vi "abort_delta.vi"() -> ()   [LabVIEW 2019]
panel:
  in  "Abort Conductance":bool
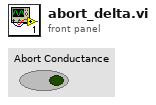
[diagram p1: front panel]
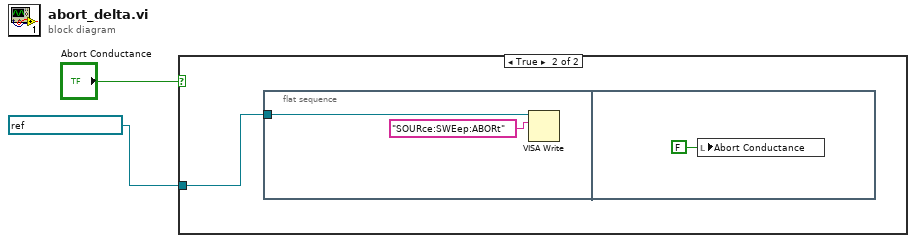
[diagram p0: block diagram]
diagram:
  n1 = case shown="True" "Abort Conductance" {
    tunnel: refnum<visa-resource-name> "GPIB1::20::INSTR" ("Keithley") -> [_ w3]
    frame False {
    }
    frame True {
      n2 = flat-sequence {
        tunnel: w3 -> [w4]
        frame #0 {
          n3 = VISA Write(VISA resource name=w4, write buffer="SOURce:SWEep:ABORt") -> ()  [unwired: 1 in, 3 out]
        }
        frame #1 {
          n4 = local write "Abort Conductance"(FALSE) -> ()
        }
      }
    }
  }
